vi "ipg_ulong.vi"(1 "String":string) -> (0 "Ulong":u32)   [LabVIEW 2019]
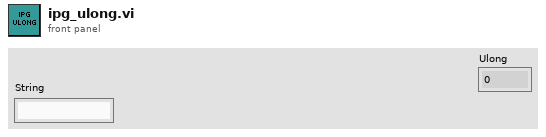
[diagram p1: front panel]
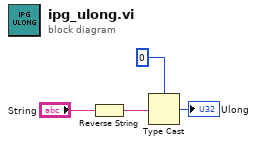
[diagram p0: block diagram]
diagram:
  n1 = Reverse String(1:"String") -> (0:w3:string)
  n2 = Type Cast(type=u32 0, x=w3) -> (*(type *) &x=→"Ulong":u32)
